vi "Stitching-Generate z-stack image path.vi"(9 "File increment number / Z-plane number":i32, 10 "Experiment folder name":string, 11 "Base directory":path) -> (3 "appended path":path)   [LabVIEW 2020]
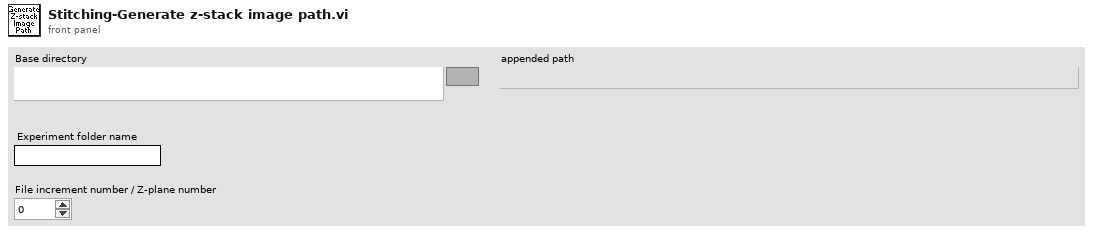
[diagram p1: front panel]
types:
  T1 = typedef "Fixed strings.ctl" = cluster{"ROI file name":string, "Normalised ROI file name":string, "Zplane Pockels values file name":string, "Functional data folder name":string, "Experiment Header file name":string, "Z-stack images folder name":string, "Groups setup rel. path":string, "Groups text file rel. path":string, "TDMS files folder name (F.img)":string, "TDMS files folder name (V.acq)":string, "TDMS files folder name (Pl.acq)":string, "Cycle rel times sequence file":string, "Dynamically called VIs folder name":string, "Time Series folder base name":string}
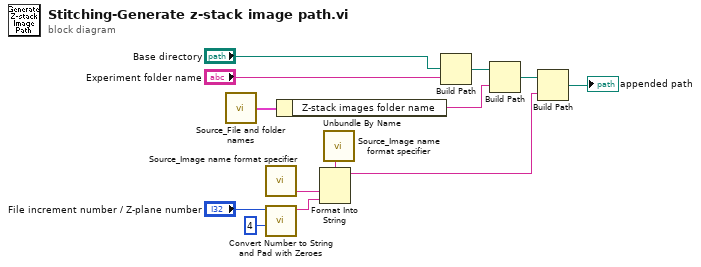
[diagram p0: block diagram]
diagram:
  n1 = call "Source_File and folder names.vi"() -> ("Fixed strings"=w2:T1)  [unwired: 1 in]
  n2 = call "Source_Image name format specifier.vi"() -> ("Green channel name"=w9:string)  [unwired: 5 in, 2 out]
  n3 = call "Convert Number to String and Pad with Zeroes.vi"("Minimum Width"=i16 4, "Number"="File increment number / Z-plane number") -> ("Number in string representation (padded with zeroes)"=w11:string)  [unwired: 9 in]
  n4 = Unbundle By Name(w2) -> ("Z-stack images folder name"=w1:string)
  n5 = call "Source_Image name format specifier.vi"() -> ("Z-Stack Image name format specifier"=w10:string)  [unwired: 5 in, 2 out]
  n6 = Format Into String(format string=w10, w9, w11) -> (resulting string=w12:string)  [unwired: 2 in, 1 out]
  n7 = Build Path(base path="Base directory", name or relative path="Experiment folder name") -> (appended path=w3:path)
  n8 = Build Path(base path=w3, name or relative path=w1) -> (appended path=w8:path)
  n9 = Build Path(base path=w8, name or relative path=w12) -> (appended path=→"appended path":path)
